vi "Buzzer_Test.vi"(8 "error in (no error)":errorcluster, 11 "Limit":string="1950~2050~0.01") -> (0 "error out":errorcluster, 2 "TestResult":bool=TRUE, 3 "TestData":string="Freq.:2003.41    AMP:0.11096")   [LabVIEW 2013]
uses:
  <vilib>/sound2/lvsound2.llb/Sampling Mode.ctl
  <vilib>/sound2/lvsound2.llb/Sound Data Format.ctl
  <vilib>/sound2/lvsound2.llb/Sound Input Read (DBL).vi
  <vilib>/measure/matone.llb/Extract Single Tone Information N Chan.vi
  <vilib>/measure/NI_MAPro.lvlib
panel:
  # "Freq.:3840.51    AMP:0.00160"
  # "NG Sample1: Freq.:4089.59    AMP:0.00059"
  # "NG Sample2: Freq.:2.42    AMP:0.00043\nFreq.:688.50    AMP:0.00311\nFreq.:709.51    AMP:0.04181"
  # "OK Sample: Freq.:770.45    AMP:0.11818"
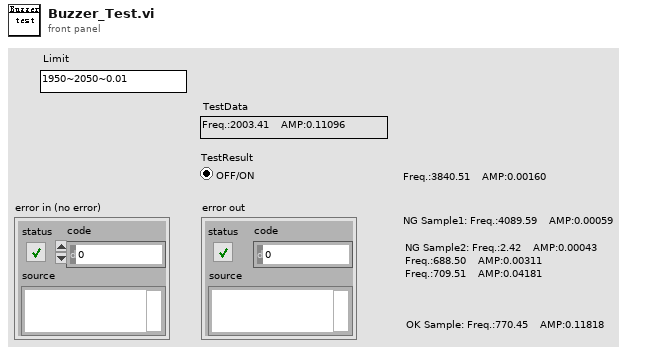
[diagram p1: front panel]
types:
  T1 = typedef "Sound Data Format.ctl" = cluster{"sample rate (S/s)":dbl, "number of channels":i32, "bits per sample":i32}
  T2 = typedef "Sampling Mode.ctl" = i32
  T3 = typedef "Sound Input Task ID.ctl" = u32
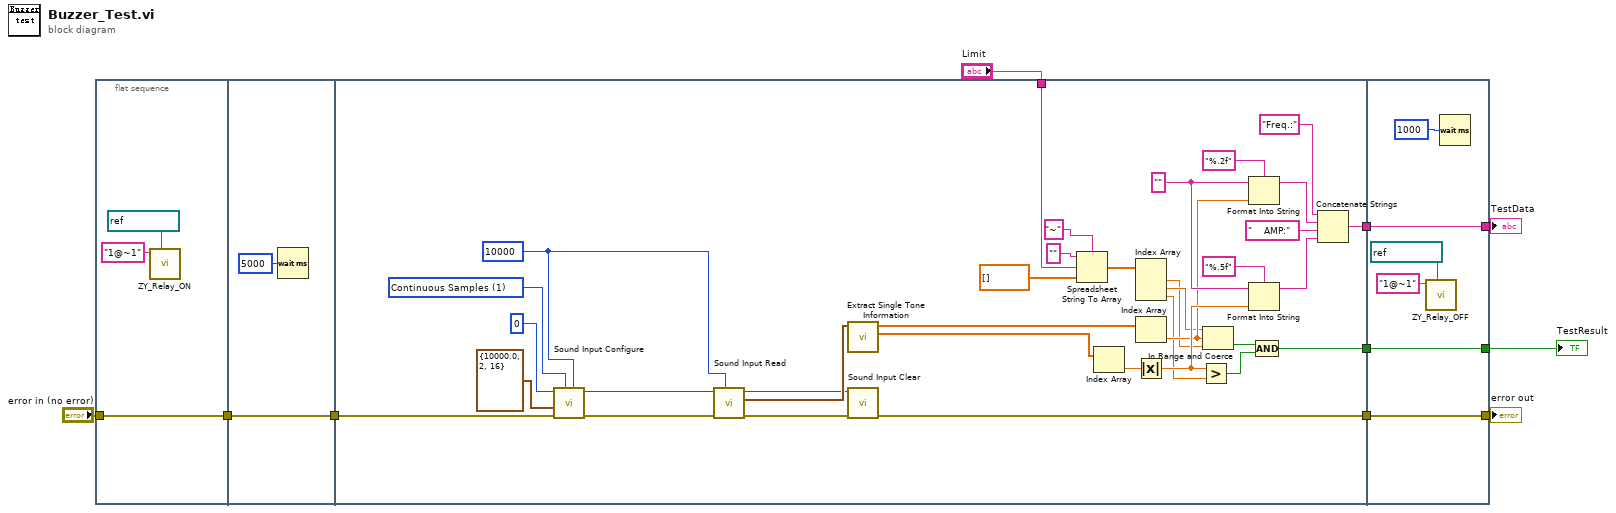
[diagram p0: block diagram]
diagram:
  n1 = flat-sequence {
    tunnel: "error in (no error)" -> [w13]
    tunnel: [w13] -> w1
    tunnel: [w15] -> w2
    tunnel: w1 -> [w15]
    tunnel: "Limit" -> [w24]
    tunnel: [w27] -> w5
    tunnel: [w26] -> w4
    tunnel: [w25] -> w3
    tunnel: w2 -> [w16]
    tunnel: [w54] -> w8
    tunnel: [w55] -> w9
    tunnel: [w56] -> w10
    tunnel: w5 -> [w56]
    tunnel: w4 -> [w55]
    tunnel: w3 -> [w54]
    frame #0 {
      n2 = call "ZY_Relay_ON.vi"("COM"=refnum<visa-resource-name> "COM22", "Limit in"="1@~1") -> ()  [unwired: 7 in, 3 out]
    }
    frame #1 {
      n3 = Wait (ms)(milliseconds to wait=u32 5000) -> ()  [unwired: 1 out]
    }
    frame #2 {
      w38 = "" ("initial string")
      w45 = 10000 ("Number of Samples/ch")
      w44 = T2 1 items=["Finite Samples", "Continuous Samples"] ("sample mode")
      n4 = call <vilib>:"Sound Input Configure.vi"("number of samples/ch"=w45, "sample mode"=w44, "error in (no error)"=w16, "sound format"=T1 {"sample rate (S/s)"=10000.0, "number of channels"=2, "bits per sample"=16} ("Sound Format"), "device ID"=u32 0 ("Device ID")) -> ("error out"=w39:errorcluster, "task ID"=w41:T3)  [unwired: 2 in, 3 out]
      n5 = call-poly <vilib>:"Sound Input Read.vi"("number of samples/ch"=w45, "error in (no error)"=w39, "task ID"=w41) -> ("error out"=w43:errorcluster, "data"=w49:waveform(dbl)[], "task ID out"=w42:T3)  [unwired: 1 in, 5 out]
      n6 = call-poly <vilib>:"Extract Single Tone Information.vi"("time signals in"=w49) -> ("detected amplitudes"=w48:dbl[], "detected frequencies"=w47:dbl[])  [unwired: 3 in, 6 out]
      n7 = call <vilib>:"Sound Input Clear.vi"("error in (no error)"=w43, "task ID"=w42) -> ("error out"=w25:errorcluster)  [unwired: 9 out]
      n8 = Spreadsheet String To Array(delimiter (Tab)="~", format string="", spreadsheet string=w24, array type (2D Dbl)=dbl[] []) -> (array=w20:dbl[])
      n9 = Index Array(array=w48) -> (element=w50:dbl)  [unwired: 1 in]
      n10 = Index Array(array=w20) -> (element #1=w18:dbl, element #2=w19:dbl, element #3=w17:dbl)  [unwired: 3 in]
      n11 = Index Array(array=w47) -> (element=w29:dbl)  [unwired: 1 in]
      n12 = Absolute Value(x=w50) -> (abs(x)=w31:dbl)
      n13 = Greater?(x=w31, y=w17) -> (0:w28:bool)
      n14 = In Range and Coerce(upper limit=w19, x=w29, lower limit=w18) -> (In Range?=w30:bool)  [unwired: 1 out]
      n15 = Format Into String(format string="%.2f", initial string=w38, w29) -> (resulting string=w36:string)  [unwired: 1 in, 1 out]
      n16 = Format Into String(format string="%.5f", initial string=w38, w31) -> (resulting string=w34:string)  [unwired: 1 in, 1 out]
      n17 = Compound Arithmetic op=AND(w30, w28) -> (w27:bool)
      n18 = Concatenate Strings("Freq.:" ("string"), w36, "    AMP:" ("string"), w34) -> (w26:string)
    }
    frame #3 {
      n19 = call "ZY_Relay_OFF.vi"("COM"=refnum<visa-resource-name> "COM22", "Limit in"="1@~1") -> ()  [unwired: 7 in, 3 out]
      n20 = Wait (ms)(milliseconds to wait=u32 1000) -> ()  [unwired: 1 out]
    }
  }
  "TestResult" <- w10
  "TestData" <- w9
  "error out" <- w8
